vi "Lift.vi"(0 "LiftLocation":T1(ring)) -> ()   [LabVIEW 2018]
uses:
  <vilib>/Rock Robotics/SystemInterfaces/DIO/FPGA_DIOChannel.ctl
  <vilib>/Rock Robotics/WPI/ThirdParty/Phoenix-LabVIEW/Motor Controller/Controls/CTRE_Phoenix_MotorControl_ControlMode.ctl
  Lift Global.vi
  Times/Times Global.vi
  <vilib>/addons/control/pid/pid.llb/PID (DBL).vi
  <vilib>/Rock Robotics/WPI/ThirdParty/Phoenix-LabVIEW/Motor Controller/Get/CTRE_Phoenix_MotorController_GetSelectedSensorData.vi
  Cargo Intake/Cargo Intake Global.vi
  <vilib>/addons/control/pid/NI_PID_pid.lvlib
panel:
  in  "Output Scalar":dbl=0.6 format="%#_13g"
  in  "t":dbl=0.6 format="%#_13g"
  in  "output range":cluster{"output high":dbl, "output low":dbl}={"output high"=1.0, "output low"=-1.0}
  in  "LiftMode":T2(ring)=enum."Basic Control"
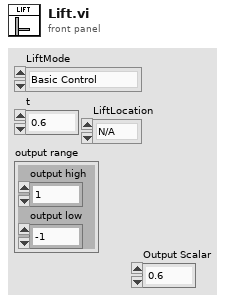
[diagram p1: front panel]
types:
  T1 = enum16{"N/A", "Hatch Panel Zone 1", "Hatch Panel Zone 2", "Hatch Panel Zone 3", "Cargo Zone 1", "Cargo Zone 2", "Cargo Zone 3"}
  T2 = enum16{"Ultra Manual Control", "Manual Control", "Basic Control", "Automated Control", "Autonomous Control"}
  T3 = typedef "FPGA_DIOChannel.ctl" = enum8{"DIO 0", "DIO 1", "DIO 2", "DIO 3", "DIO 4", "DIO 5", "DIO 6", "DIO 7", "DIO 8", "DIO 9", "DIO MXP 0", "DIO MXP 1", "DIO MXP 2", "DIO MXP 3", "DIO MXP 4", "DIO MXP 5", "DIO MXP 6", "DIO MXP 7", "DIO MXP 8", "DIO MXP 9", "DIO MXP 10", "DIO MXP 11", "DIO MXP 12", "DIO MXP 13", "DIO MXP 14", "DIO MXP 15", "SPI Port CS1", "SPI Port CS2", "SPI Port CS3", "SPI Port MISO", "SPI Port MOSI", "Invalid"}
  T4 = typedef "WPI_DigitalInputDevRef.ctl" = cluster{"DevStatus":errorcluster, "DIO Channel":T3}
  T5 = typedef "WPI_MotorControlDeviceRef.ctl" = cluster{"DeviceStatus":errorcluster, "Type":T6, "PWM":cluster{"PWM Channel":T7, "DeadBand":T8}, "CAN":cluster{"Device Number":u8, "SetOutput VI Ref":variant, "GetOutput VI Ref":variant, "Enable VI Ref":variant, "Disable VI Ref":variant, "Data":variant}, "Invert":bool, "DIO PWM":cluster{"PWM \"Enable\" Channel":T7, "DIOChannel":T3, "PWM Rate":dbl}}
  T6 = typedef "WPI_MotorControlType.ctl" = enum16{"PWM", "CAN", "DIO PWM"}
  T7 = typedef "FPGA_DIOPWMChannel.ctl" = enum8{"PWM 0", "PWM 1", "PWM 2", "PWM 3", "PWM 4", "PWM 5", "PWM 6", "PWM 7", "PWM 8", "PWM 9", "PWM MXP 0", "PWM MXP 1", "PWM MXP 2", "PWM MXP 3", "PWM MXP 4", "PWM MXP 5", "PWM MXP 6", "PWM MXP 7", "PWM MXP 8", "PWM MXP 9", "Invalid"}
  T8 = typedef "WPI_PWMDeadband.ctl" = cluster{"Name":string, "maxPositivePwm":i32, "minPositivePwm":i32, "centerPwm":i32, "maxNegativePwm":i32, "minNegativePwm":i32, "angularRange":u16}
  T9 = typedef "CTRE_Phoenix_MotorControl_ControlMode.ctl" = u16
  T10 = cluster{"proportional gain (Kc)":dbl, "integral time(Ti, min)":dbl, "derivative time(Td, min) 2":dbl}
  T11 = enum16{"Hatch Panel Zone 1", "Hatch Panel Zone 2", "Hatch Panel Zone 3", "Cargo Zone 1", "Cargo Zone 2", "Cargo Zone 3", "Cargo Ship Zone"}
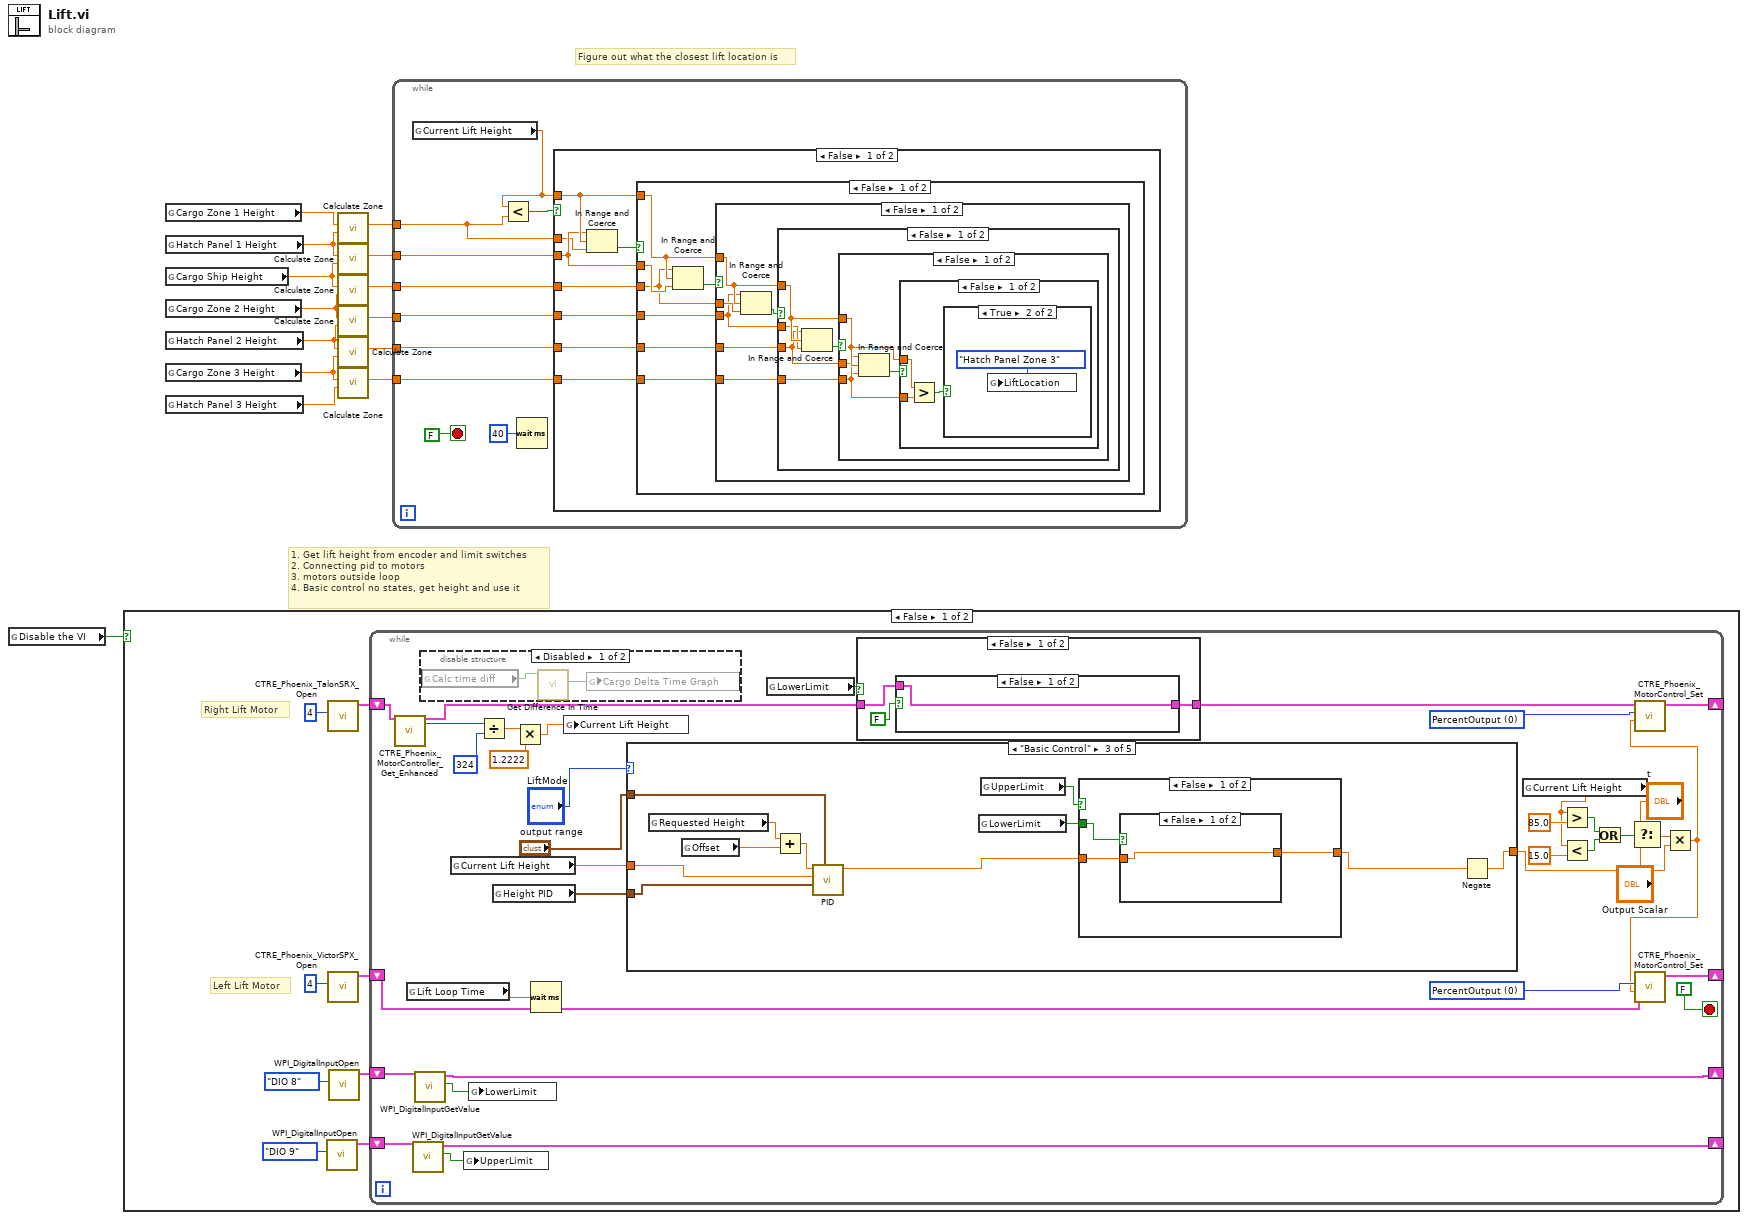
[diagram p0: block diagram]
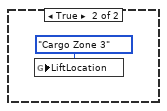
[diagram p3: hidden frame]
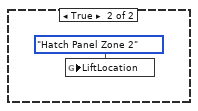
[diagram p4: hidden frame]
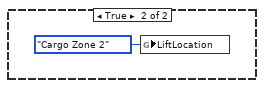
[diagram p5: hidden frame]
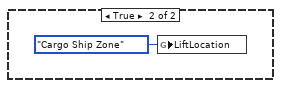
[diagram p6: hidden frame]
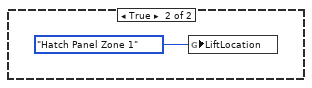
[diagram p7: hidden frame]
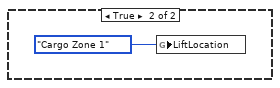
[diagram p8: hidden frame]
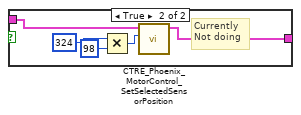
[diagram p9: hidden frame]
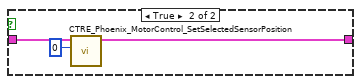
[diagram p10: hidden frame]
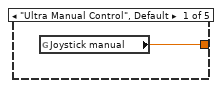
[diagram p12: hidden frame]
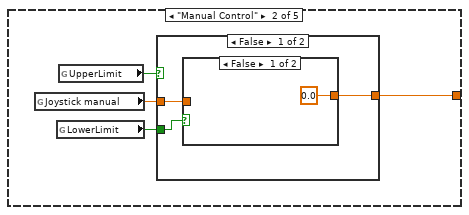
[diagram p13: hidden frame]
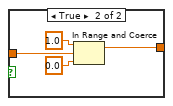
[diagram p14: hidden frame]
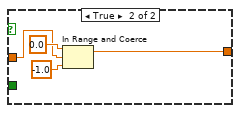
[diagram p15: hidden frame]
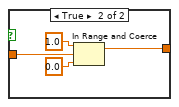
[diagram p16: hidden frame]
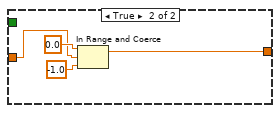
[diagram p17: hidden frame]
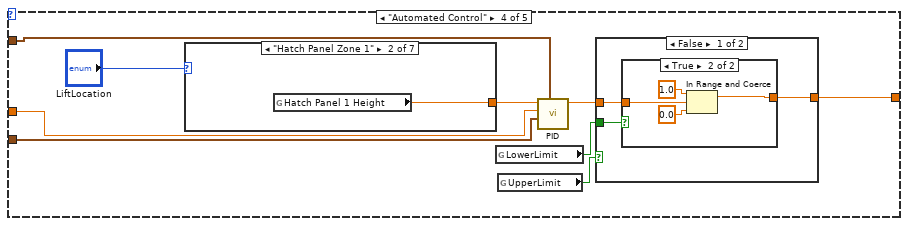
[diagram p18: hidden frame]
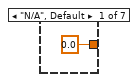
[diagram p19: hidden frame]
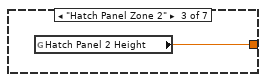
[diagram p20: hidden frame]
diagram:
  # "Figure out what the closest lift location is"
  # "1. Get lift height from encoder and limit switches\n2. Connecting pid to motors\n3. motors outside loop\n4. Basic control no states, get height and use it"
  n1 = global read "Lift Global.vi" "Disable the VI"() -> (w14:bool)
  n2 = case shown="False" w14 {
    frame False {
      # "Left Lift Motor"
      # "Right Lift Motor"
      n3 = call <vilib>:"WPI_DigitalInputOpen.vi"("DIO Channel"=FPGA_DIOChannel."DIO 9") -> ("DigitalInputDevRef"=w15:T4)  [unwired: 9 in, 1 out]
      n4 = call <vilib>:"CTRE_Phoenix_TalonSRX_Open.vi"("Device Number"=u8 4) -> ("CAN Talon SRX Ref"=w22:T5)  [unwired: 9 in, 1 out]
      n5 = call <vilib>:"CTRE_Phoenix_VictorSPX_Open.vi"("Device Number"=u8 4) -> ("CAN Talon SRX Ref"=w20:T5)  [unwired: 9 in, 1 out]
      n6 = call <vilib>:"WPI_DigitalInputOpen.vi"("DIO Channel"=FPGA_DIOChannel."DIO 8") -> ("DigitalInputDevRef"=w17:T4)  [unwired: 9 in, 1 out]
      n7 = while {
        shift-right: [w55] -> _
        shift-left: w22 -> [w48]
        shift-right: [w53] -> _
        shift-left: w20 -> [w52]
        shift-right: [w42] -> _
        shift-left: w17 -> [w43]
        shift-right: [w37] -> _
        shift-left: w15 -> [w38]
        stop <- FALSE stop-if-true
        w54 = T9 0 items=["PercentOutput"=0, "Position"=1, "Velocity"=2, "Current"=3, "Follower"=5, "MotionProfile"=6, "MotionMagic"=7, "MotionProfileArc"=10, "Disabled"=15] ("Control Mode")
        w56 = T9 0 items=["PercentOutput"=0, "Position"=1, "Velocity"=2, "Current"=3, "Follower"=5, "MotionProfile"=6, "MotionMagic"=7, "MotionProfileArc"=10, "Disabled"=15] ("Control Mode")
        n8 = call-poly <vilib>:"CTRE_Phoenix_MotorController_Get_Enhanced.vi"("PhoenixMotorControlDevRef"=w48) -> ("PhoenixMotorControlDevRef"=w47:T5, "Position (Raw Sensor Units)"=w45:i32)  [unwired: 11 in, 2 out]
        n9 = global read "Times Global.vi" "Lift Loop Time"() -> (w59:dbl)
        n10 = call <vilib>:"WPI_DigitalInputGetValue.vi"("DigitalInputDevRef"=w38) -> ("Value"=w40:bool, "DigitalInputDevRef"=w37:T4)  [unwired: 8 in, 1 out]
        n11 = call <vilib>:"WPI_DigitalInputGetValue.vi"("DigitalInputDevRef"=w43) -> ("Value"=w41:bool, "DigitalInputDevRef"=w42:T4)  [unwired: 8 in, 1 out]
        n12 = disable-structure shown="Disabled" {
          frame Disabled {
            n13 = global read "Cargo Intake Global.vi" "Calc time diff"() -> (w73:bool)
            n14 = call "Get Difference In Time.vi"("Calculate Time Difference"=w73) -> ("Delta Time over Time"=w72:u32)  [unwired: 9 in, 1 out]
            n15 = global write "Times Global.vi" "Cargo Delta Time Graph"(w72) -> ()
          }
          frame Enabled {
          }
        }
        n16 = global read "Lift Global.vi" "Current Lift Height"() -> (w49:dbl)
        n17 = global write "Lift Global.vi" "UpperLimit"(w40) -> ()
        n18 = global write "Lift Global.vi" "LowerLimit"(w41) -> ()
        n19 = Divide(x=w45, y=324) -> (x/y=w25:dbl)
        n20 = global read "Lift Global.vi" "Height PID"() -> (w50:T10)
        n21 = Multiply(x=w25, y=1.2222) -> (x*y=w24:dbl)
        n22 = Wait (ms)(milliseconds to wait=w59) -> ()  [unwired: 1 out]
        n23 = global write "Lift Global.vi" "Current Lift Height"(w24) -> ()
        n24 = case shown="\"Basic Control\"" "LiftMode" {
          tunnel: [w74 w75 w98 w119 0.0 ("Cargo Zone 3 Height")] -> w29
          tunnel: w49 -> [_ _ w101 w117 _]
          tunnel: w50 -> [_ _ w100 w116 _]
          tunnel: "output range" -> [_ _ w99 w118 _]
          frame "Ultra Manual Control", Default {
            n25 = global read "Lift Global.vi" "Joystick manual"() -> (w74:dbl)
          }
          frame "Manual Control" {
            n26 = global read "Lift Global.vi" "Joystick manual"() -> (w76:dbl)
            n27 = global read "Lift Global.vi" "LowerLimit"() -> (w78:bool)
            n28 = global read "Lift Global.vi" "UpperLimit"() -> (w77:bool)
            n29 = case shown="False" w77 {
              tunnel: w78 -> [w81 _]
              tunnel: [w80 w88] -> w75
              tunnel: w76 -> [w79 w87]
              frame False {
                n30 = case shown="False" w81 {
                  tunnel: [0.0 w86] -> w80
                  tunnel: w79 -> [_ w83]
                  frame False {
                  }
                  frame True {
                    n31 = In Range and Coerce(upper limit=1.0, x=w83, lower limit=0.0) -> (coerced(x)=w86:dbl)  [unwired: 1 out]
                  }
                }
              }
              frame True {
                n32 = In Range and Coerce(upper limit=0.0, x=w87, lower limit=-1.0) -> (coerced(x)=w88:dbl)  [unwired: 1 out]
              }
            }
          }
          frame "Basic Control" {
            n33 = global read "Lift Global.vi" "Requested Height"() -> (w91:dbl)
            n34 = global read "Lift Global.vi" "Offset"() -> (w92:dbl)
            n35 = Add(x=w91, y=w92) -> (x+y=w93:dbl)
            n36 = call-poly <vilib>:"PID.vi"("output range"=w99, "PID gains"=w100, "process variable"=w101, "setpoint"=w93) -> ("output"=w95:dbl)  [unwired: 6 in, 1 out]
            n37 = global read "Lift Global.vi" "LowerLimit"() -> (w97:bool)
            n38 = global read "Lift Global.vi" "UpperLimit"() -> (w96:bool)
            n39 = case shown="False" w96 {
              tunnel: w97 -> [w104 _]
              tunnel: [w103 w111] -> w94
              tunnel: w95 -> [w102 w110]
              frame False {
                n40 = case shown="False" w104 {
                  tunnel: [w105 w109] -> w103
                  tunnel: w102 -> [w105 w106]
                  frame False {
                  }
                  frame True {
                    n41 = In Range and Coerce(upper limit=1.0, x=w106, lower limit=0.0) -> (coerced(x)=w109:dbl)  [unwired: 1 out]
                  }
                }
              }
              frame True {
                n42 = In Range and Coerce(upper limit=0.0, x=w110, lower limit=-1.0) -> (coerced(x)=w111:dbl)  [unwired: 1 out]
              }
            }
            n43 = Negate(x=w94) -> (-x=w98:dbl)
          }
          frame "Automated Control" {
            n44 = case shown="\"Hatch Panel Zone 1\"" "LiftLocation" {
              tunnel: [0.0 ("Cargo Zone 3 Height") w124 w125 w126 w127 w128 w129] -> w114
              frame "N/A", Default {
              }
              frame "Hatch Panel Zone 1" {
                n45 = global read "Lift Global.vi" "Hatch Panel 1 Height"() -> (w124:dbl)
              }
              frame "Hatch Panel Zone 2" {
                n46 = global read "Lift Global.vi" "Hatch Panel 2 Height"() -> (w125:dbl)
              }
              frame "Hatch Panel Zone 3" {
                n47 = global read "Lift Global.vi" "Hatch Panel 3 Height"() -> (w126:dbl)
              }
              frame "Cargo Zone 1" {
                n48 = global read "Lift Global.vi" "Cargo Zone 1 Height"() -> (w127:dbl)
              }
              frame "Cargo Zone 2" {
                n49 = global read "Lift Global.vi" "Cargo Zone 2 Height"() -> (w128:dbl)
              }
              frame "Cargo Zone 3" {
                n50 = global read "Lift Global.vi" "Cargo Zone 3 Height"() -> (w129:dbl)
              }
            }
            n51 = global read "Lift Global.vi" "LowerLimit"() -> (w122:bool)
            n52 = global read "Lift Global.vi" "UpperLimit"() -> (w121:bool)
            n53 = call-poly <vilib>:"PID.vi"("output range"=w118, "PID gains"=w116, "process variable"=w117, "setpoint"=w114) -> ("output"=w120:dbl)  [unwired: 6 in, 1 out]
            n54 = case shown="False" w121 {
              tunnel: w122 -> [w132 _]
              tunnel: [w131 w139] -> w119
              tunnel: w120 -> [w130 w138]
              frame False {
                n55 = case shown="True" w132 {
                  tunnel: [0.0 w137] -> w131
                  tunnel: w130 -> [_ w134]
                  frame False {
                  }
                  frame True {
                    n56 = In Range and Coerce(upper limit=1.0, x=w134, lower limit=0.0) -> (coerced(x)=w137:dbl)  [unwired: 1 out]
                  }
                }
              }
              frame True {
                n57 = In Range and Coerce(upper limit=0.0, x=w138, lower limit=-1.0) -> (coerced(x)=w139:dbl)  [unwired: 1 out]
              }
            }
          }
          frame "Autonomous Control" {
          }
        }
        n58 = global read "Lift Global.vi" "LowerLimit"() -> (w39:bool)
        n59 = case shown="False" w39 {
          tunnel: w47 -> [w62 w71]
          tunnel: [w61 w70] -> w46
          frame False {
            n60 = case shown="False" FALSE {
              tunnel: w62 -> [w63 w68]
              tunnel: [w63 w67] -> w61
              frame False {
              }
              frame True {
                # "Currently\nNot doing"
                n61 = Multiply(x=324 ("y"), y=98 ("New Sensor Position")) -> (x*y=w64:i32)
                n62 = call <vilib>:"CTRE_Phoenix_MotorControl_SetSelectedSensorPosition.vi"("New Sensor Position"=w64, "PhoenixMotorControlDevRef"=w68) -> ("PhoenixMotorControlDevRef"=w67:T5)  [unwired: 8 in, 1 out]
              }
            }
          }
          frame True {
            n63 = call <vilib>:"CTRE_Phoenix_MotorControl_SetSelectedSensorPosition.vi"("New Sensor Position"=0, "PhoenixMotorControlDevRef"=w71) -> ("PhoenixMotorControlDevRef"=w70:T5)  [unwired: 8 in, 1 out]
          }
        }
        n64 = global read "Lift Global.vi" "Current Lift Height"() -> (w34:dbl)
        n65 = Greater?(x=w34, y=85.0) -> (0:w32:bool)
        n66 = Less?(x=w34, y=15.0) -> (x < y?=w33:bool)
        n67 = Or(x=w32, y=w33) -> (x .or. y?=w31:bool)
        n68 = Select(t="t", s=w31, f="Output Scalar") -> (s? t:f=w30:dbl)
        n69 = Multiply(x=w30, y=w29) -> (x*y=w26:dbl)
        n70 = call <vilib>:"CTRE_Phoenix_MotorControl_Set.vi"("Output"=w26, "Control Mode"=w56, "PhoenixMotorControlDevRef"=w46) -> ("PhoenixMotorControlDevRef"=w55:T5)  [unwired: 7 in, 1 out]
        n71 = call <vilib>:"CTRE_Phoenix_MotorControl_Set.vi"("Output"=w26, "Control Mode"=w54, "PhoenixMotorControlDevRef"=w52) -> ("PhoenixMotorControlDevRef"=w53:T5)  [unwired: 7 in, 1 out]
      }
    }
    frame True {
    }
  }
  n72 = global read "Lift Global.vi" "Cargo Zone 1 Height"() -> (w7:dbl)
  n73 = global read "Lift Global.vi" "Hatch Panel 1 Height"() -> (w13:dbl)
  n74 = global read "Lift Global.vi" "Cargo Ship Height"() -> (w12:dbl)
  n75 = global read "Lift Global.vi" "Cargo Zone 2 Height"() -> (w11:dbl)
  n76 = global read "Lift Global.vi" "Hatch Panel 2 Height"() -> (w10:dbl)
  n77 = global read "Lift Global.vi" "Cargo Zone 3 Height"() -> (w9:dbl)
  n78 = global read "Lift Global.vi" "Hatch Panel 3 Height"() -> (w8:dbl)
  n79 = call "Calculate Zone.vi"("Top Height"=w13, "Bottom Height"=w7) -> ("Midpoint"=w6:dbl)  [unwired: 9 in]
  n80 = call "Calculate Zone.vi"("Top Height"=w12, "Bottom Height"=w13) -> ("Midpoint"=w5:dbl)  [unwired: 9 in]
  n81 = call "Calculate Zone.vi"("Top Height"=w11, "Bottom Height"=w12) -> ("Midpoint"=w4:dbl)  [unwired: 9 in]
  n82 = call "Calculate Zone.vi"("Top Height"=w10, "Bottom Height"=w11) -> ("Midpoint"=w3:dbl)  [unwired: 9 in]
  n83 = call "Calculate Zone.vi"("Top Height"=w9, "Bottom Height"=w10) -> ("Midpoint"=w2:dbl)  [unwired: 9 in]
  n84 = call "Calculate Zone.vi"("Top Height"=w8, "Bottom Height"=w9) -> ("Midpoint"=w1:dbl)  [unwired: 9 in]
  n85 = while {
    tunnel: w6 -> [w148]
    tunnel: w5 -> [w147]
    tunnel: w4 -> [w146]
    tunnel: w3 -> [w145]
    tunnel: w2 -> [w144]
    tunnel: w1 -> [w143]
    stop <- FALSE stop-if-true
    n86 = global read "Lift Global.vi" "Current Lift Height"() -> (w149:dbl)
    n87 = Less?(x=w149, y=w148) -> (x < y?=w150:bool)
    n88 = Wait (ms)(milliseconds to wait=u32 40) -> ()  [unwired: 1 out]
    n89 = case shown="False" w150 {
      tunnel: w149 -> [w156 _]
      tunnel: w148 -> [w154 _]
      tunnel: w147 -> [w155 _]
      tunnel: w146 -> [w160 _]
      tunnel: w145 -> [w159 _]
      tunnel: w144 -> [w158 _]
      tunnel: w143 -> [w157 _]
      frame False {
        n90 = In Range and Coerce(upper limit=w155, x=w156, lower limit=w154) -> (In Range?=w153:bool)  [unwired: 1 out]
        n91 = case shown="False" w153 {
          tunnel: w156 -> [w163 _]
          tunnel: w155 -> [w162 _]
          tunnel: w160 -> [w161 _]
          tunnel: w159 -> [w167 _]
          tunnel: w158 -> [w166 _]
          tunnel: w157 -> [w165 _]
          frame False {
            n92 = In Range and Coerce(upper limit=w161, x=w163, lower limit=w162) -> (In Range?=w164:bool)  [unwired: 1 out]
            n93 = case shown="False" w164 {
              tunnel: w163 -> [w170 _]
              tunnel: w167 -> [w168 _]
              tunnel: w166 -> [w173 _]
              tunnel: w165 -> [w172 _]
              tunnel: w161 -> [w169 _]
              frame False {
                n94 = In Range and Coerce(upper limit=w168, x=w170, lower limit=w169) -> (In Range?=w171:bool)  [unwired: 1 out]
                n95 = case shown="False" w171 {
                  tunnel: w170 -> [w176 _]
                  tunnel: w173 -> [w174 _]
                  tunnel: w172 -> [w178 _]
                  tunnel: w168 -> [w175 _]
                  frame False {
                    n96 = In Range and Coerce(upper limit=w174, x=w176, lower limit=w175) -> (In Range?=w177:bool)  [unwired: 1 out]
                    n97 = case shown="False" w177 {
                      tunnel: w176 -> [w181 _]
                      tunnel: w178 -> [w180 _]
                      tunnel: w174 -> [w179 _]
                      frame False {
                        n98 = In Range and Coerce(upper limit=w180, x=w181, lower limit=w179) -> (In Range?=w182:bool)  [unwired: 1 out]
                        n99 = case shown="False" w182 {
                          tunnel: w181 -> [w185 _]
                          tunnel: w180 -> [w184 _]
                          frame False {
                            n100 = Greater?(x=w185, y=w184) -> (0:w183:bool)
                            n101 = case shown="True" w183 {
                              frame False {
                              }
                              frame True {
                                n102 = global write "Lift Global.vi" "LiftLocation"(T11."Hatch Panel Zone 3" ("LiftLocation")) -> ()
                              }
                            }
                          }
                          frame True {
                            n103 = global write "Lift Global.vi" "LiftLocation"(T11."Cargo Zone 3" ("LiftLocation")) -> ()
                          }
                        }
                      }
                      frame True {
                        n104 = global write "Lift Global.vi" "LiftLocation"(T11."Hatch Panel Zone 2" ("LiftLocation")) -> ()
                      }
                    }
                  }
                  frame True {
                    n105 = global write "Lift Global.vi" "LiftLocation"(T11."Cargo Zone 2" ("LiftLocation")) -> ()
                  }
                }
              }
              frame True {
                n106 = global write "Lift Global.vi" "LiftLocation"(T11."Cargo Ship Zone" ("LiftLocation")) -> ()
              }
            }
          }
          frame True {
            n107 = global write "Lift Global.vi" "LiftLocation"(T11."Hatch Panel Zone 1" ("LiftLocation")) -> ()
          }
        }
      }
      frame True {
        n108 = global write "Lift Global.vi" "LiftLocation"(T11."Cargo Zone 1" ("LiftLocation")) -> ()
      }
    }
  }
